vi "Create Message Setter (from Accessor).vi"(8 "error in (no error)":errorcluster, 10 "RPC Message Name":string, 11 "RPC Messages Folder (ProjectItem) in":refnum<vi>) -> (0 "error out":errorcluster, 1 "Created ?":bool, 2 "Getter VI out":refnum<vi>, 3 "RPC Messages Folder (ProjectItem) out":refnum<vi>)   [LabVIEW 2019, in "gRPC Scripting Tools.lvlib"]
uses:
  gRPC Scripting Tools.lvlib
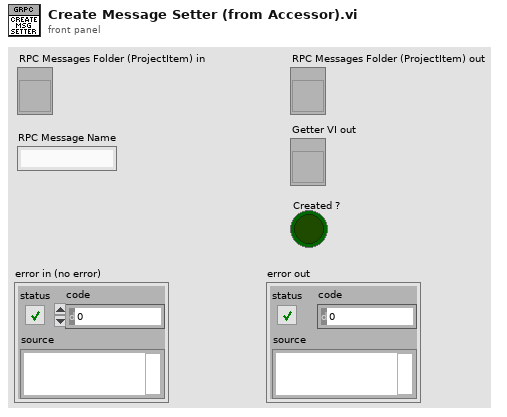
[diagram p1: front panel]
types:
  T1 = enum32{"invalid VI type", "Standard VI", "Control VI", "Global VI", "Polymorphic VI", "Configuration VI", "SubSystem", "Facade VI", "Method VI"}
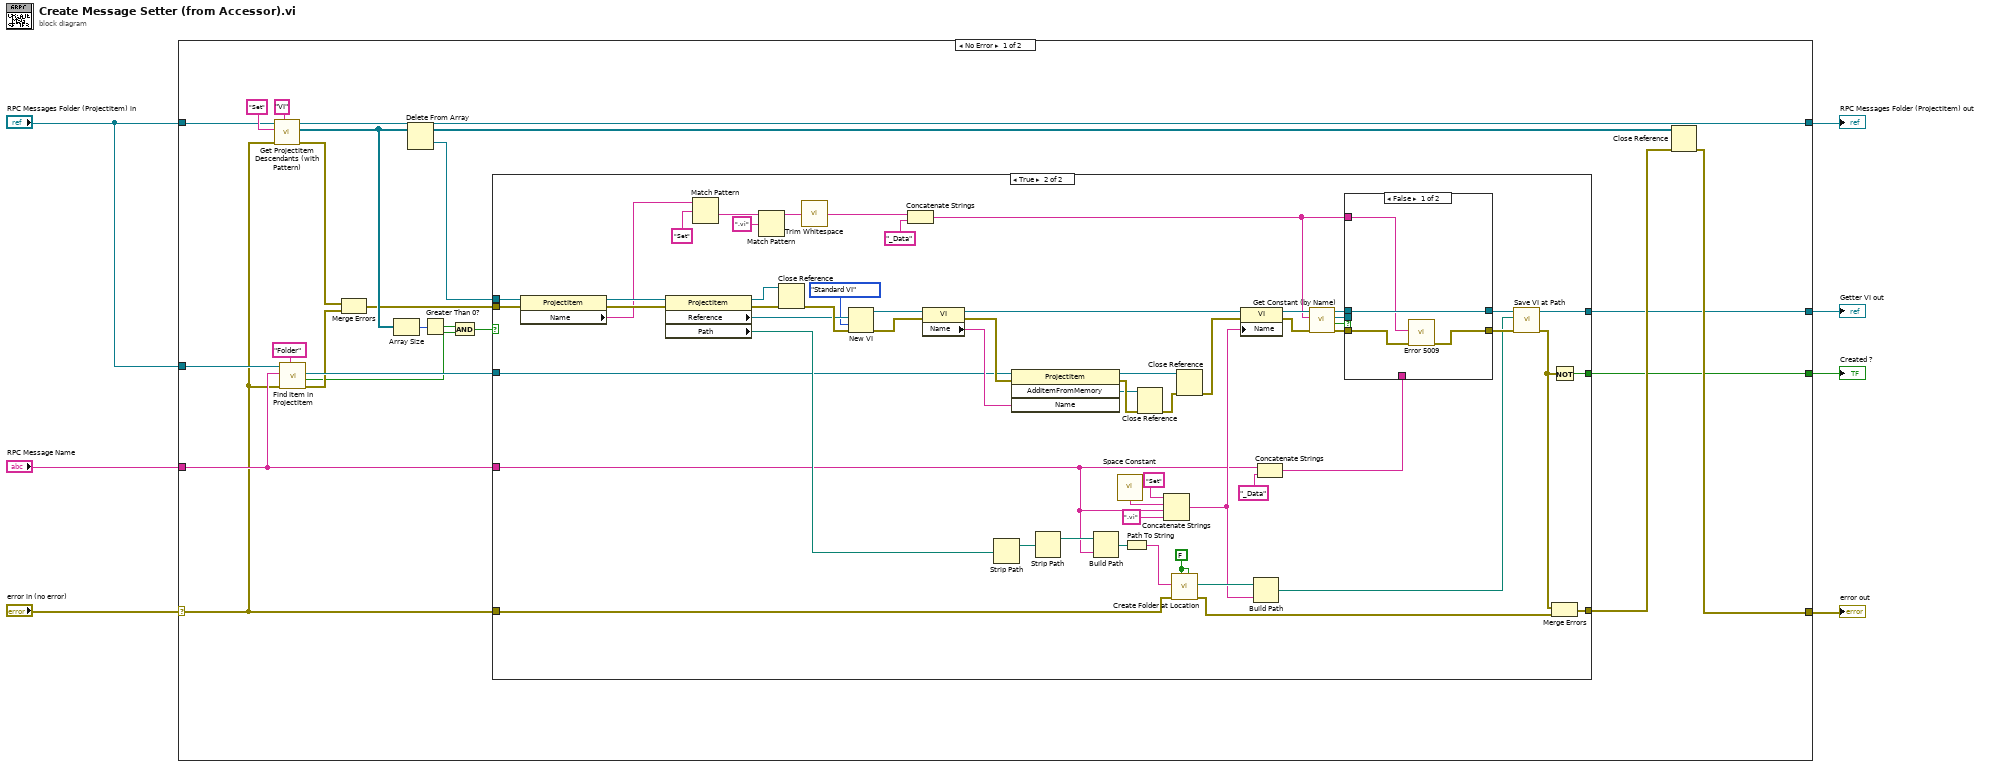
[diagram p0: block diagram]
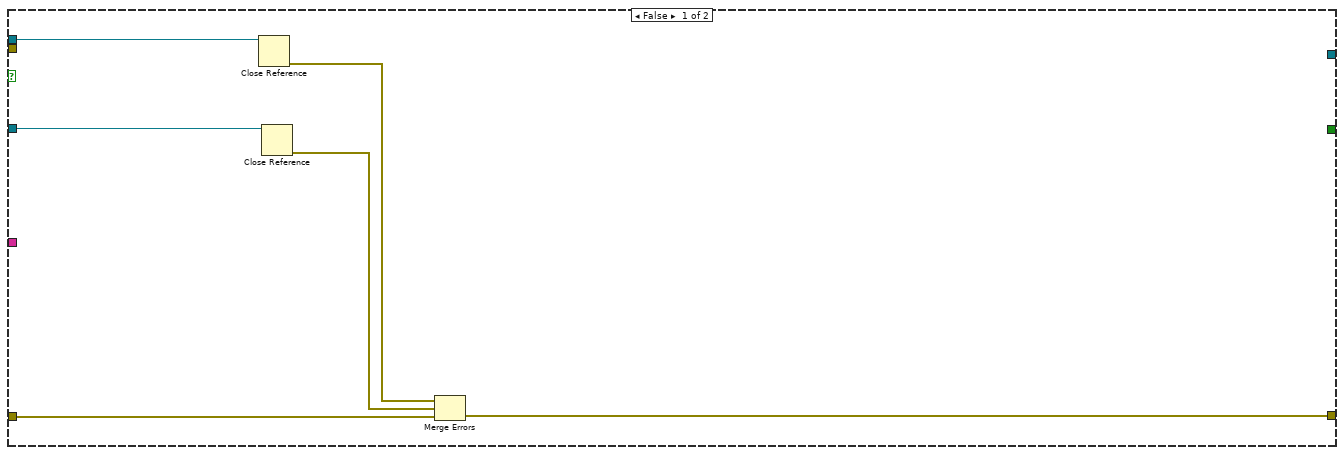
[diagram p2: hidden frame]
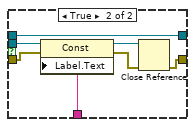
[diagram p3: hidden frame]
diagram:
  n1 = case shown="No Error" "error in (no error)" {
    selector: "error in (no error)" -> [w13 w106]
    tunnel: "RPC Message Name" -> [w25 _]
    tunnel: "RPC Messages Folder (ProjectItem) in" -> [w23 _]
    tunnel: "RPC Messages Folder (ProjectItem) in" -> [w18 w105]
    tunnel: [w11 w106] -> w4
    tunnel: [w10 w105] -> w3
    tunnel: [w9 _] -> w2
    tunnel: [w8 _] -> w1
    frame No Error {
      n2 = call "Get ProjectItem Descendants (with Pattern).vi"("Type"="VI", "error in (no error)"=w13, "Pattern"="Set", "ProjectItem in"=w18) -> ("error out"=w17:errorcluster, "ProjectItem descendents"=w24:refnum<vi>[], "ProjectItem out"=w10:refnum<vi>)  [unwired: 5 in]
      n3 = call "Find Item in ProjectItem.vi"("Item Type"="Folder", "error in (no error)"=w13, "Name"=w25, "ProjectItem in"=w23) -> ("error out"=w16:errorcluster, "Found ?"=w15:bool, "Item Refnum out"=w21:refnum<vi>)  [unwired: 4 in, 1 out]
      n4 = Merge Errors(w17, w16) -> (w14:errorcluster)
      n5 = Array Size(array=w24) -> (size(s)=w22:i32)
      n6 = Delete From Array(array=w24) -> (deleted portion=w27:refnum<vi>, array with subset deleted=w30:refnum<vi>[])  [unwired: 2 in]
      n7 = Greater Than 0?(x=w22) -> (x > 0?=w20:bool)
      n8 = And(x=w20, y=w15) -> (x .and. y?=w19:bool)
      n9 = case shown="True" w19 {
        tunnel: w25 -> [_ w48]
        tunnel: [w33 w90] -> w12
        tunnel: [_ w44] -> w8
        tunnel: w27 -> [w36 w62]
        tunnel: [_ w72] -> w9
        tunnel: w21 -> [w31 w67]
        tunnel: w13 -> [w32 w66]
        tunnel: w14 -> [_ w61]
        frame False {
          n10 = Close Reference(reference=w36) -> (error out=w34:errorcluster)  [unwired: 1 in]
          n11 = Close Reference(reference=w31) -> (error out=w35:errorcluster)  [unwired: 1 in]
          n12 = Merge Errors(w34, w35, w32) -> (w33:errorcluster)
        }
        frame True {
          w88 = FALSE ("Use Relative (F)")
          n13 = property class="ProjectItem"(reference=w62, error in=w61) -> (reference out=w60:refnum<vi>, error out=w59:errorcluster, "Name"=w58:string)
          n14 = property class="ProjectItem"(reference=w60, error in=w59) -> (reference out=w93:refnum<vi>, error out=w91:errorcluster, "Reference"=w78:refnum<vi>, "Path"=w84:path)
          n15 = Match Pattern(string=w58, regular expression="Set") -> (after substring=w56:string)  [unwired: 1 in, 3 out]
          n16 = Match Pattern(string=w56, regular expression=".vi") -> (before substring=w41:string)  [unwired: 1 in, 3 out]
          n17 = Close Reference(reference=w93, error in (no error)=w91) -> (error out=w92:errorcluster)
          n18 = call <vilib>:"Trim Whitespace.vi"("string"=w41) -> ("trimmed string"=w54:string)  [unwired: 1 in]
          n19 = New VI(8:w92, 9:T1."Standard VI" ("vi type (standard vi)"), 10:w78) -> (0:w77:errorcluster, 3:w75:refnum<vi>)  [unwired: 1 in, 3 out]
          n20 = Concatenate Strings(w54, "_Data" ("string")) -> (w37:string)
          n21 = property class="VI"(reference=w75, error in=w77) -> (reference out=w85:refnum<vi>, error out=w86:errorcluster, "Name"=w79:string)
          n22 = Strip Path(path=w84) -> (stripped path=w80:path)  [unwired: 1 out]
          n23 = invoke class="ProjectItem" method="AddItemFromMemory"(reference=w67, error in=w86, "Name"=w79) -> (reference out=w74:refnum<vi>, error out=w65:errorcluster, "AddItemFromMemory"=w64:refnum<vi>)  [unwired: 1 in, 1 out]
          n24 = Strip Path(path=w80) -> (stripped path=w81:path)  [unwired: 1 out]
          n25 = Build Path(base path=w81, name or relative path=w48) -> (appended path=w82:path)
          n26 = call <vilib>:"Space Constant.vi"() -> ("String"=w70:string)
          n27 = Path To String(path=w82) -> (string=w83:string)
          n28 = Close Reference(reference=w64, error in (no error)=w65) -> (error out=w63:errorcluster)
          n29 = Concatenate Strings("Set" ("string"), w70, w48, ".vi" ("string")) -> (w68:string)
          n30 = call "Create Folder at Location.vi"("Override existing (F)"=w88, "Use Relative (F)"=w88, "Error In"=w66, "Path"=w83) -> ("Error Out"=w89:errorcluster, "Full path out"=w87:path)  [unwired: 5 in, 1 out]
          n31 = Close Reference(reference=w74, error in (no error)=w63) -> (error out=w73:errorcluster)
          n32 = property class="VI"(reference=w85, error in=w73, "Name"=w68) -> (reference out=w51:refnum<vi>, error out=w50:errorcluster)
          n33 = Build Path(base path=w87, name or relative path=w68) -> (appended path=w43:path)
          n34 = Concatenate Strings(w48, "_Data" ("string")) -> (w47:string)
          n35 = call "Get Constant (by Name).vi"("error in (no error)"=w50, "Constant Label"=w37, "Owner VI in"=w51) -> ("error out"=w46:errorcluster, "Found ?"=w40:bool, "Const ref out"=w52:refnum<vi>, "Owner VI out"=w39:refnum<vi>)  [unwired: 5 in]
          n36 = case shown="False" w40 {
            tunnel: w52 -> [_ w104]
            tunnel: w47 -> [_ w103]
            tunnel: w46 -> [w96 w102]
            tunnel: [w95 w99] -> w45
            tunnel: w39 -> [w97 w98]
            tunnel: [w97 w98] -> w38
            tunnel: w37 -> [w94 _]
            frame False {
              n37 = call "Error 5009.vi"("error in (no error)"=w96, "Cluster Definition Constant"=w94) -> ("error out"=w95:errorcluster)  [unwired: 9 in]
            }
            frame True {
              n38 = property class="Const"(reference=w104, error in=w102, "Label.Text"=w103) -> (reference out=w101:refnum<vi>, error out=w100:errorcluster)
              n39 = Close Reference(reference=w101, error in (no error)=w100) -> (error out=w99:errorcluster)
            }
          }
          n40 = call "Save VI at Path.vi"("error in (no error)"=w45, "Path"=w43, "VI in"=w38) -> ("error out"=w42:errorcluster, "VI out"=w44:refnum<vi>)  [unwired: 6 in, 1 out]
          n41 = Not(x=w42) -> (.not. x?=w72:bool)
          n42 = Merge Errors(w42, w89) -> (w90:errorcluster)
        }
      }
      n43 = Close Reference(reference=w30, error in (no error)=w12) -> (error out=w11:errorcluster)
    }
    frame Error {
    }
  }
  "error out" <- w4
  "RPC Messages Folder (ProjectItem) out" <- w3
  "Created ?" <- w2
  "Getter VI out" <- w1
